vi "Count up to 17575 with 3 Characters.vi"(1 "Numeric Control":i32) -> (0 "string":string)   [LabVIEW 2015]
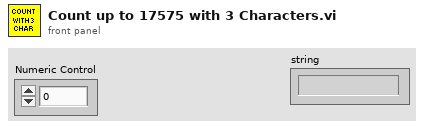
[diagram p1: front panel]
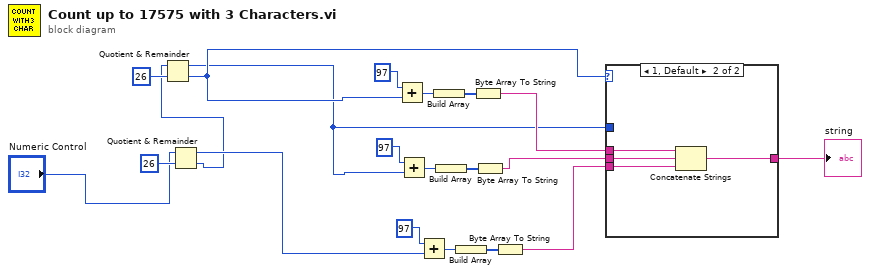
[diagram p0: block diagram]
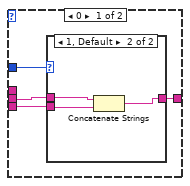
[diagram p2: hidden frame]
diagram:
  n1 = Quotient & Remainder(x="Numeric Control", y=26) -> (x-y*floor(x/y)=w4:i32, floor(x/y)=w2:i32)
  n2 = Quotient & Remainder(x=w2, y=26) -> (x-y*floor(x/y)=w1:i32, floor(x/y)=w3:i32)
  n3 = Add(x=97, y=w3) -> (x+y=w9:i32)
  n4 = Add(x=97, y=w1) -> (x+y=w12:i32)
  n5 = Add(x=97, y=w4) -> (x+y=w15:i32)
  n6 = Build Array(w9) -> (w10:i32[])
  n7 = Build Array(w12) -> (w11:i32[])
  n8 = Build Array(w15) -> (w16:i32[])
  n9 = Byte Array To String(unsigned byte array=w10) -> (string=w7:string)
  n10 = Byte Array To String(unsigned byte array=w11) -> (string=w6:string)
  n11 = Byte Array To String(unsigned byte array=w16) -> (string=w5:string)
  n12 = case shown="1, Default" w3 {
    tunnel: [w23 w32] -> w17
    tunnel: w7 -> [_ w31]
    tunnel: w6 -> [w21 w30]
    tunnel: w5 -> [w22 w29]
    tunnel: w1 -> [w24 _]
    frame 0 {
      n13 = case shown="1, Default" w24 {
        tunnel: [w25 w26] -> w23
        tunnel: w22 -> [w25 w27]
        tunnel: w21 -> [_ w28]
        frame 0 {
        }
        frame 1, Default {
          n14 = Concatenate Strings(w28, w27) -> (w26:string)
        }
      }
    }
    frame 1, Default {
      n15 = Concatenate Strings(w31, w30, w29) -> (w32:string)
    }
  }
  "string" <- w17
